vi "MTMount_cancelCallback_command_standby.vi"(8 "error in (no error)":errorcluster) -> (0 "error out":errorcluster, 3 "function return":i32)   [LabVIEW 2018, in "SALLV_MTMount.lvlib"]
doc: "int MTMount_shm_cancelCallback_command_standbyLV();"
uses:
  SALLV_MTMount.lvlib
  SALLV_MTMount.so
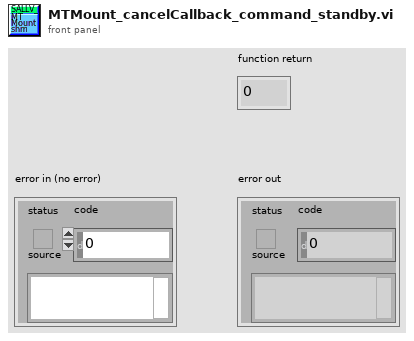
[diagram p1: front panel]
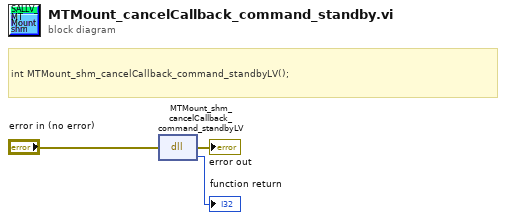
[diagram p0: block diagram]
diagram:
  # "int MTMount_shm_cancelCallback_command_standbyLV();"
  n1 = dll-call lib="home/ttsai/Document/salApiMTMount/SALLV_MTMount/SALLV_MTMount.*" fn="MTMount_shm_cancelCallback_command_standbyLV"(error in="error in (no error)") -> (error out=→"error out":errorcluster, →"function return":i32)  [unwired: 2 in, 1 out]
